vi "Constant trim.vi"(11 "String":string) -> (0 "Array of Names":string[](array[string]), 3 "Array of Numbers":string[](array[string]))   [LabVIEW 2013]
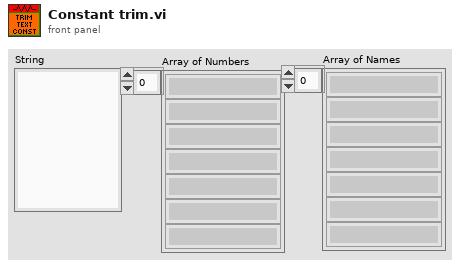
[diagram p1: front panel]
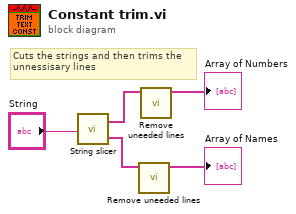
[diagram p0: block diagram]
diagram:
  # "Cuts the strings and then trims the\nunnessisary lines"
  n1 = call "String slicer.vi"("Multiline String"="String") -> ("Array of numbers with spaces"=w4:string[], "Array of variable names"=w2:string[])
  n2 = call "Remove uneeded lines.vi"("Array"=w2) -> ("Array out"=→"Array of Names":string[])  [unwired: 10 in]
  n3 = call "Remove uneeded lines.vi"("Array"=w4) -> ("Array out"=→"Array of Numbers":string[])  [unwired: 10 in]
